vi "Untitled 2 (SubVI).vi"(11 "trimmed string":string) -> (3 "Numeric":dbl)   [LabVIEW 2017]
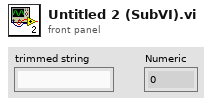
[diagram p1: front panel]
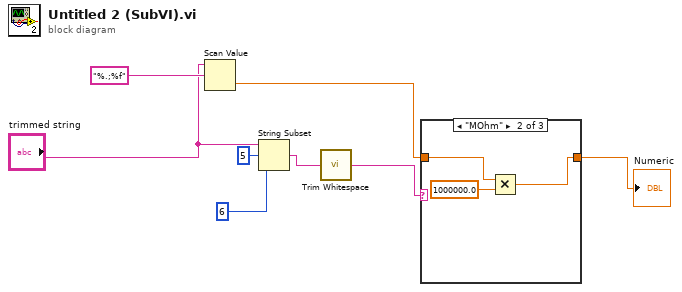
[diagram p0: block diagram]
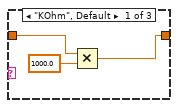
[diagram p2: hidden frame]
diagram:
  n1 = Scan Value(string="trimmed string", format string="%.;%f") -> (value=w2:dbl)  [unwired: 1 in, 1 out]
  n2 = String Subset(string="trimmed string", offset (0)=5, length (rest)=6 ("length (rest)")) -> (substring=w4:string)
  n3 = call <vilib>:"Trim Whitespace.vi"("string"=w4) -> ("trimmed string"=w3:string)  [unwired: 1 in]
  n4 = case shown="\"MOhm\"" w3 {
    tunnel: [w9 w12 w15] -> w1
    tunnel: w2 -> [w10 w13 w15]
    frame "KOhm", Default {
      n5 = Multiply(x=w10, y=1000.0) -> (x*y=w9:dbl)
    }
    frame "MOhm" {
      n6 = Multiply(x=w13, y=1000000.0) -> (x*y=w12:dbl)
    }
    frame "Ohm" {
    }
  }
  "Numeric" <- w1
